vi "面积.vi"(8 "error in (no error)":errorcluster caption="错误输入（无错误）", 11 "封闭形状 输入":refnum<class "封闭形状.lvclass"> caption="DNL_LabVIEW Object in") -> (0 "error out":errorcluster caption="错误输出", 2 "面积":dbl, 3 "封闭形状 输出":refnum<class "封闭形状.lvclass"> caption="DNL_LabVIEW Object out")   [LabVIEW 2013, in "封闭形状.lvclass"]
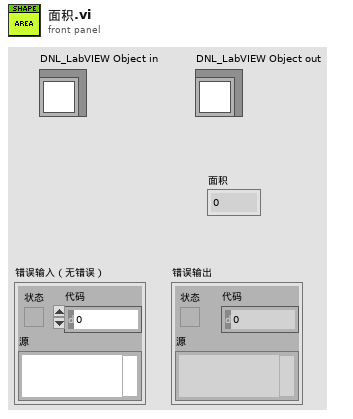
[diagram p1: front panel]
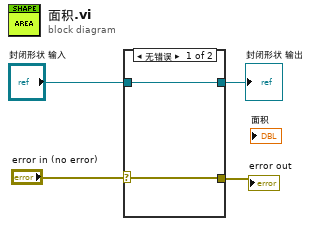
[diagram p0: block diagram]
diagram:
  n1 = case shown="无错误" "error in (no error)" {
    selector: "error in (no error)" -> [w5 w8]
    tunnel: [w5 w8] -> w3
    tunnel: [w6 w7] -> w1
    tunnel: "封闭形状 输入" -> [w6 w7]
    frame No Error {
    }
    frame Error {
    }
  }
  "error out" <- w3
  "封闭形状 输出" <- w1
